vi "LoadHexaSummary1.vi"(7 "Machine":string, 10 "file path (dialog if empty)":path=path "C:/m300/HEXA/R141201634_20141222_141239.lot") -> (0 "error out":errorcluster)   [LabVIEW 2012]
uses:
  <vilib>/Utility/miscctls.llb/LVDateTimeRec.ctl
  <vilib>/addons/database/Auxilliary.llb/DB Tools Cursor Type.ctl
  <vilib>/addons/database/Connection.llb/DB Tools Open Connec (Path).vi
  <vilib>/addons/database/Connection.llb/Conn Execute.vi
  <vilib>/addons/database/Recordset.llb/Rec Fetch Integer Data (R).vi
  <vilib>/addons/database/Recordset.llb/Rec Destroy - Connection.vi
  <vilib>/addons/database/NI_Database_API.lvlib
panel:
  in  "Cluster 2":T1
  out "array":string[][](array[string])
  out "concatenated string":string
  in  "date time rec":T2
  in  "Cluster":T3
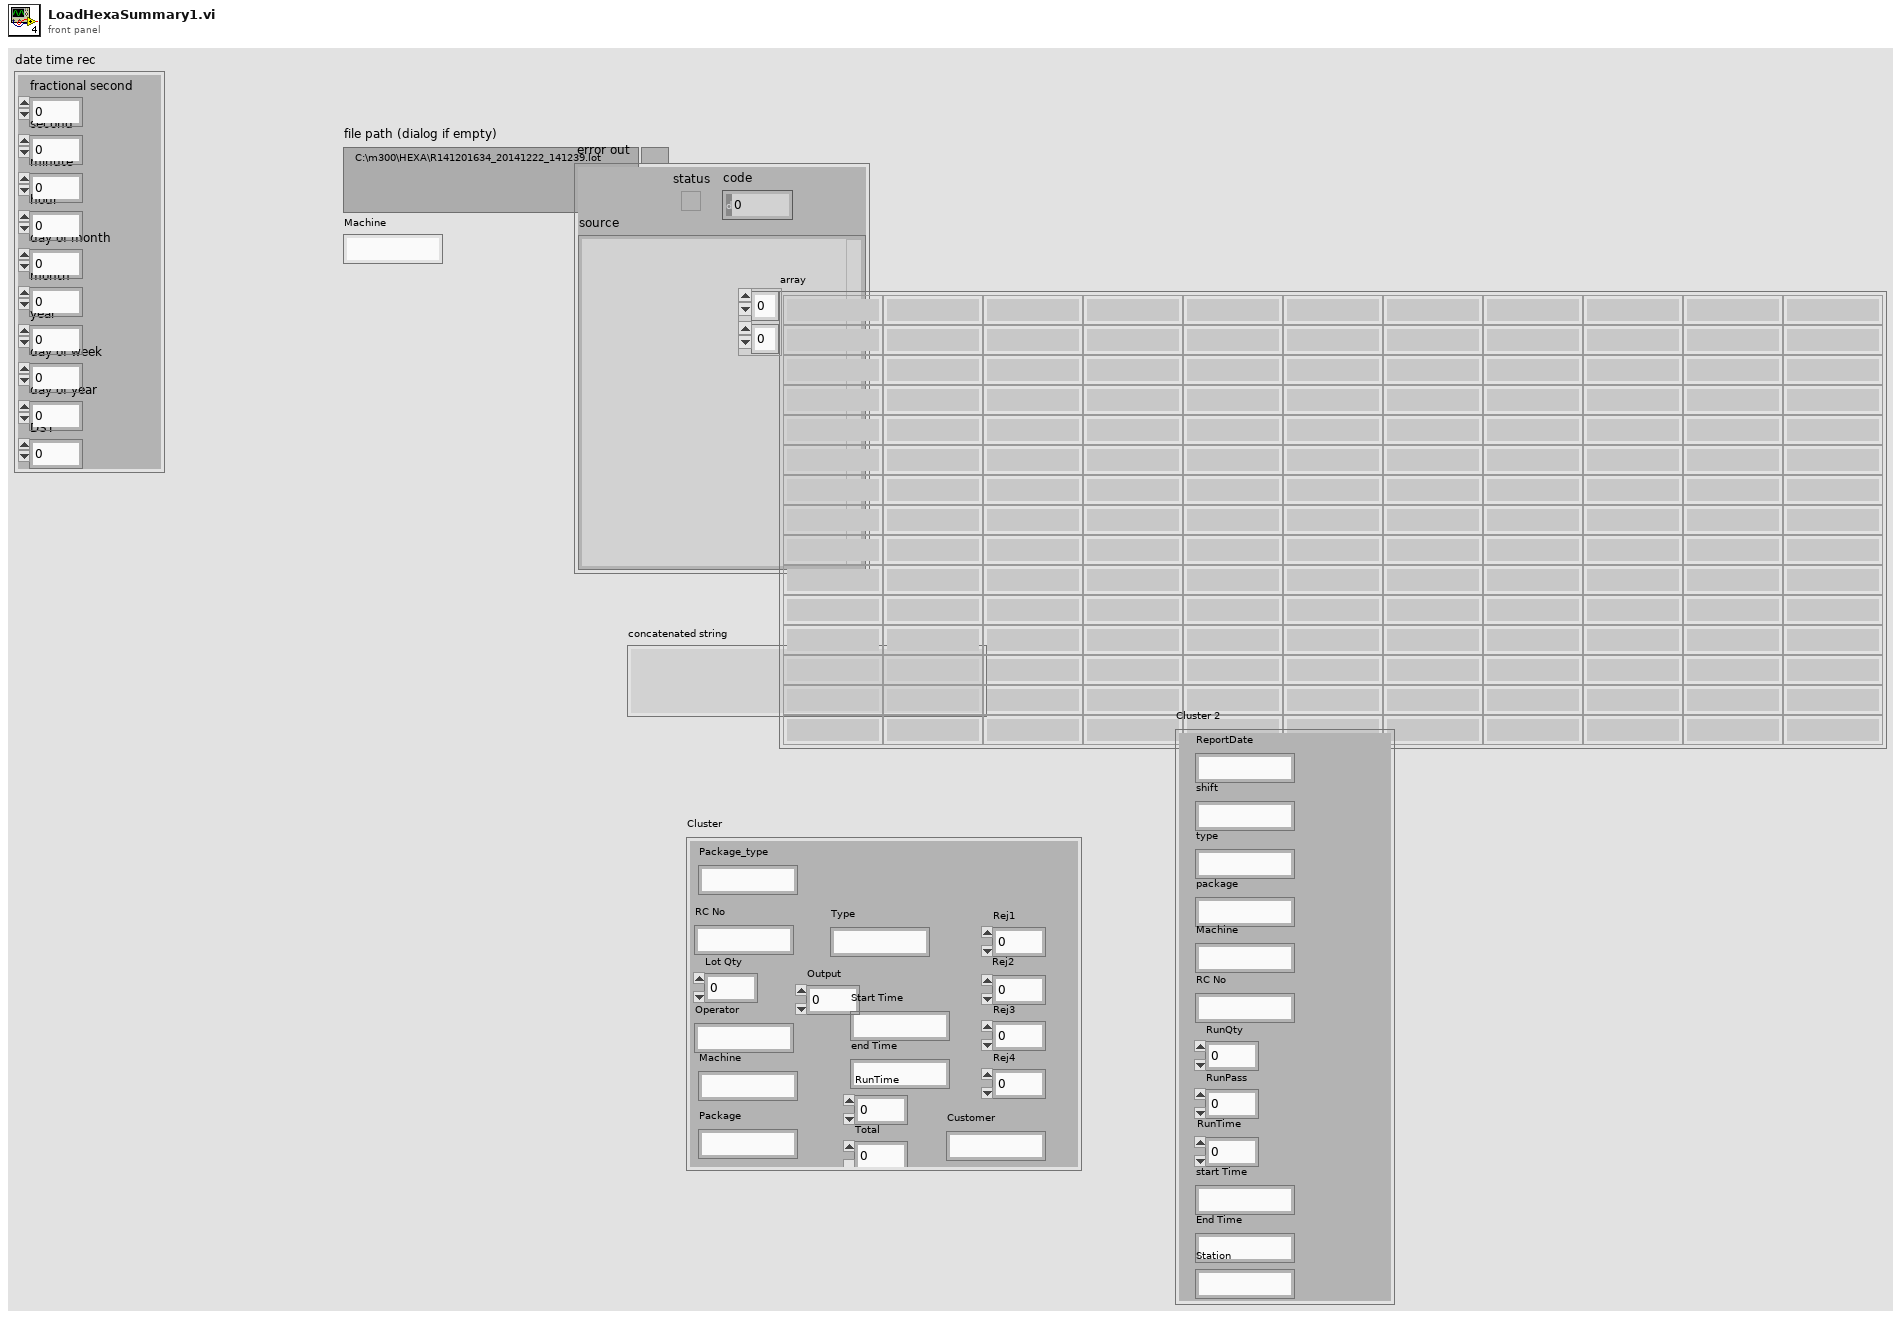
[diagram p1: front panel]
types:
  T1 = cluster{"ReportDate":string, "shift":string, "type":string, "package":string, "Machine":string, "RC No":string, "RunQty":dbl, "RunPass":dbl, "RunTime":dbl, "start Time":string, "End Time":string, "Station":string}
  T2 = typedef "LVDateTimeRec.ctl" = cluster{"fractional second":dbl, "second":i32, "minute":i32, "hour":i32, "day of month":i32, "month":i32, "year":i32, "day of week":i32, "day of year":i32, "DST":i32}
  T3 = cluster{"Package_type":string, "RC No":string, "Lot Qty":dbl, "Operator":string, "Machine":string, "Package":string, "Type":string, "Output":dbl, "Start Time":string, "end Time":string, "RunTime":dbl, "Total":dbl, "Rej1":dbl, "Rej2":dbl, "Rej3":dbl, "Rej4":dbl, "Customer":string}
  T4 = typedef "NI_Database_API.lvlib/DB Tools Cursor Type.ctl" = enum16{"forward-only", "keyset", "dynamic", "static"}
  T5 = typedef "NI_Database_API.lvlib/Conn ObjectReference.ctl" = refnum<k1>
  T6 = typedef "NI_Database_API.lvlib/Rec ObjectReference.ctl" = refnum<k1>
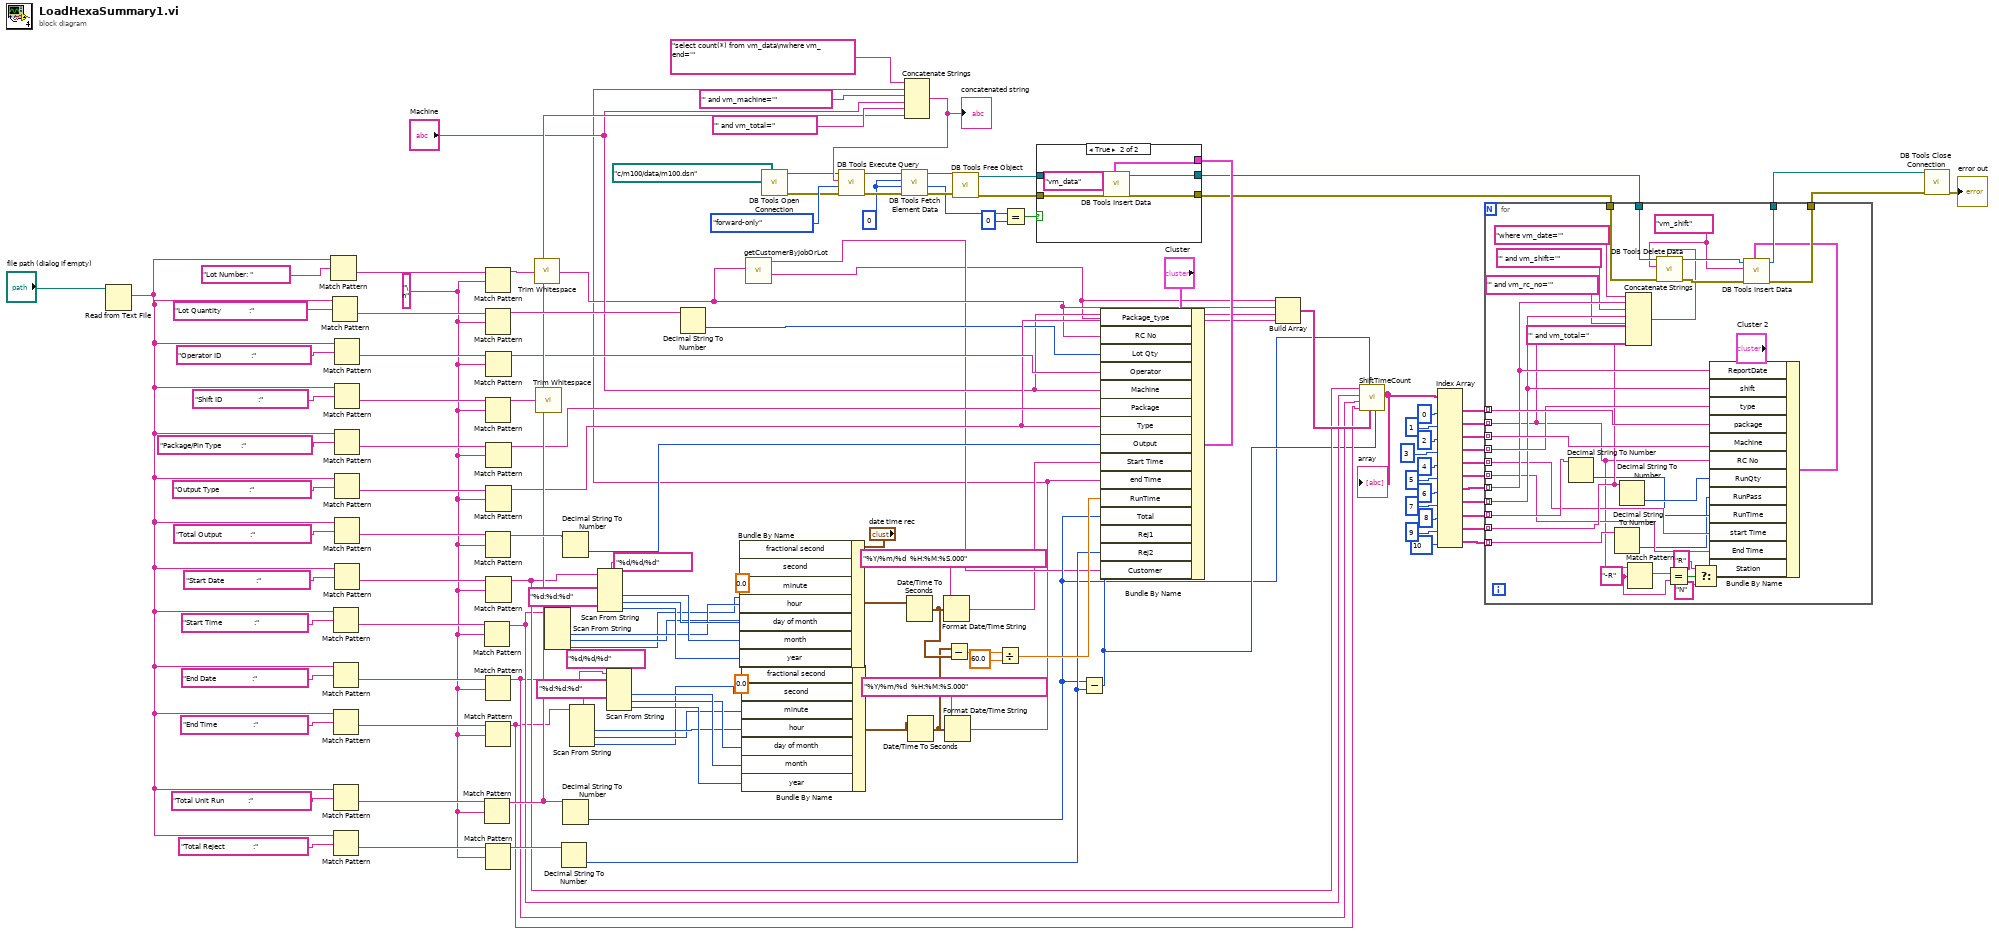
[diagram p0: block diagram]
diagram:
  w61 = 0
  w102 = "\n" ("regular expression")
  n1 = Read from Text File(file (use dialog)="file path (dialog if empty)") -> (text=w101:string)  [unwired: 3 in, 3 out]
  n2 = Match Pattern(string=w101, regular expression="Lot Number: ") -> (after substring=w127:string)  [unwired: 1 in, 3 out]
  n3 = Match Pattern(string=w101, regular expression="Lot Quantity              :") -> (after substring=w126:string)  [unwired: 1 in, 3 out]
  n4 = Match Pattern(string=w101, regular expression="Start Time                :") -> (after substring=w110:string)  [unwired: 1 in, 3 out]
  n5 = Match Pattern(string=w101, regular expression="End Date                  :") -> (after substring=w109:string)  [unwired: 1 in, 3 out]
  n6 = Match Pattern(string=w101, regular expression="End Time                  :") -> (after substring=w107:string)  [unwired: 1 in, 3 out]
  n7 = Match Pattern(string=w101, regular expression="Total Unit Run            :") -> (after substring=w104:string)  [unwired: 1 in, 3 out]
  n8 = Match Pattern(string=w101, regular expression="Total Reject              :") -> (after substring=w103:string)  [unwired: 1 in, 3 out]
  n9 = Match Pattern(string=w101, regular expression="Operator ID               :") -> (after substring=w123:string)  [unwired: 1 in, 3 out]
  n10 = Match Pattern(string=w101, regular expression="Shift ID                  :") -> (after substring=w120:string)  [unwired: 1 in, 3 out]
  n11 = Match Pattern(string=w101, regular expression="Package/Pin Type          :") -> (after substring=w119:string)  [unwired: 1 in, 3 out]
  n12 = Match Pattern(string=w101, regular expression="Output Type               :") -> (after substring=w117:string)  [unwired: 1 in, 3 out]
  n13 = Match Pattern(string=w101, regular expression="Total Output              :") -> (after substring=w114:string)  [unwired: 1 in, 3 out]
  n14 = Match Pattern(string=w101, regular expression="Start Date                :") -> (after substring=w113:string)  [unwired: 1 in, 3 out]
  n15 = Match Pattern(string=w110, regular expression=w102) -> (before substring=w38:string)  [unwired: 1 in, 3 out]
  n16 = Match Pattern(string=w104, regular expression=w102) -> (before substring=w47:string)  [unwired: 1 in, 3 out]
  n17 = Match Pattern(string=w127, regular expression=w102) -> (before substring=w54:string)  [unwired: 1 in, 3 out]
  n18 = Match Pattern(string=w126, regular expression=w102) -> (before substring=w125:string)  [unwired: 1 in, 3 out]
  n19 = Match Pattern(string=w120, regular expression=w102) -> (before substring=w53:string)  [unwired: 1 in, 3 out]
  n20 = Match Pattern(string=w114, regular expression=w102) -> (before substring=w100:string)  [unwired: 1 in, 3 out]
  n21 = Match Pattern(string=w109, regular expression=w102) -> (before substring=w37:string)  [unwired: 1 in, 3 out]
  n22 = Match Pattern(string=w107, regular expression=w102) -> (before substring=w36:string)  [unwired: 1 in, 3 out]
  n23 = Match Pattern(string=w103, regular expression=w102) -> (before substring=w72:string)  [unwired: 1 in, 3 out]
  n24 = Match Pattern(string=w123, regular expression=w102) -> (before substring=w45:string)  [unwired: 1 in, 3 out]
  n25 = Match Pattern(string=w119, regular expression=w102) -> (before substring=w46:string)  [unwired: 1 in, 3 out]
  n26 = Match Pattern(string=w117, regular expression=w102) -> (before substring=w44:string)  [unwired: 1 in, 3 out]
  n27 = Match Pattern(string=w113, regular expression=w102) -> (before substring=w39:string)  [unwired: 1 in, 3 out]
  n28 = call <vilib>:"Trim Whitespace.vi"("string"=w54) -> ("trimmed string"=w5:string)  [unwired: 1 in]
  n29 = call <vilib>:"Trim Whitespace.vi"("string"=w53) -> ()  [unwired: 1 in, 1 out]
  n30 = Scan From String(format string="%d:%d:%d", input string=w38) -> (output 1=w94:i32, output 2=w93:i32, output 3=w92:i32)  [unwired: 5 in, 3 out]
  n31 = Decimal String To Number(string=w72) -> (number=w70:i32)  [unwired: 2 in, 1 out]
  n32 = Decimal String To Number(string=w100) -> (number=w73:i32)  [unwired: 2 in, 1 out]
  n33 = Decimal String To Number(string=w47) -> (number=w6:i32)  [unwired: 2 in, 1 out]
  n34 = Scan From String(format string="%d:%d:%d", input string=w36) -> (output 1=w84:i32, output 2=w83:i32, output 3=w82:i32)  [unwired: 5 in, 3 out]
  n35 = Scan From String(format string="%d/%d/%d", input string=w39) -> (output 1=w98:i32, output 2=w97:i32, output 3=w96:i32)  [unwired: 5 in, 3 out]
  n36 = Scan From String(format string="%d/%d/%d", input string=w37) -> (output 1=w87:i32, output 2=w86:i32, output 3=w85:i32)  [unwired: 5 in, 3 out]
  n37 = Decimal String To Number(string=w125) -> (number=w41:i32)  [unwired: 2 in, 1 out]
  n38 = Bundle By Name(cluster="date time rec", "fractional second"=0.0, "second"=w92, "minute"=w93, "hour"=w94, "day of month"=w97, "month"=w98, "year"=w96) -> (w80:T2)
  n39 = Bundle By Name(cluster="date time rec", "fractional second"=0.0, "second"=w82, "minute"=w83, "hour"=w84, "day of month"=w86, "month"=w87, "year"=w85) -> (w77:T2)
  n40 = call "getCustomerByJobOrLot.vi"("Lot"=w5) -> ("Package"=w3:string, "CustomerID"=w4:string)  [unwired: 9 in]
  n41 = call-poly <vilib>:"DB Tools Open Connection.vi"("connection information"=path "c:/m100/data/m100.dsn") -> ("error out"=w50:errorcluster, "connection reference"=w51:T5)  [unwired: 7 in]
  n42 = Date/Time To Seconds(2:w80) -> (0:w43:timestamp)  [unwired: 1 in]
  n43 = Date/Time To Seconds(2:w77) -> (0:w42:timestamp)  [unwired: 1 in]
  n44 = Format Date/Time String(time format string (%c)="%Y/%m/%d  %H:%M:%S.000", seconds (now)=w43) -> (date/time string=w2:string)  [unwired: 1 in]
  n45 = Format Date/Time String(time format string (%c)="%Y/%m/%d  %H:%M:%S.000", seconds (now)=w42) -> (date/time string=w1:string)  [unwired: 1 in]
  n46 = Concatenate Strings("select count(*) from vm_data\nwhere vm_end='" ("SQL query"), w1, "' and vm_machine='" ("string"), "Machine", "' and vm_total=" ("string"), w47) -> (w52:string)
  "concatenated string" <- w52
  n47 = call-poly <vilib>:"DB Tools Execute Query.vi"("error in (no error)"=w50, "cursor type"=DB_Tools_Cursor_Type."forward-only", "SQL query"=w52, "connection reference"=w51) -> ("error out"=w67:errorcluster, "recordset reference"=w69:T6)  [unwired: 4 in]
  n48 = call-poly <vilib>:"DB Tools Fetch Element Data.vi"("error in (no error)"=w67, "type"=w61, "column index"=w61, "recordset reference"=w69) -> ("error out"=w66:errorcluster, "data"=w60:i32, "recordset reference out"=w68:T6)  [unwired: 3 in]
  n49 = Subtract(x=w42, y=w43) -> (x-y=w76:dbl)
  n50 = call-poly <vilib>:"DB Tools Free Object.vi"("error in (no error)"=w66, "recordset reference"=w68) -> ("error out"=w56:errorcluster, "connection reference"=w57:T5)  [unwired: 8 in]
  n51 = Divide(x=w76, y=60.0) -> (x/y=w71:dbl)
  n52 = Equal?(x=w60, y=0) -> (x = y?=w58:bool)
  n53 = Subtract(x=w6, y=w70) -> (x-y=w7:i32)
  n54 = Bundle By Name(cluster="Cluster", "Package_type"=w3, "RC No"=w5, "Lot Qty"=w41, "Operator"=w45, "Machine"="Machine", "Package"=w46, "Type"=w44, "Output"=w73, "Start Time"=w2, "end Time"=w1, "RunTime"=w71, "Total"=w6, "Rej1"=w7, "Rej2"=w70, "Customer"=w4) -> (w55:T3)
  n55 = case shown="True" w58 {
    tunnel: w57 -> [w132 w138]
    tunnel: w56 -> [w131 w137]
    tunnel: [w132 w136] -> w13
    tunnel: [w131 w135] -> w12
    tunnel: w55 -> [_ w134]
    frame False {
    }
    frame True {
      n56 = call <vilib>:"DB Tools Insert Data.vi"("data"=w134, "error in (no error)"=w137, "table"="vm_data", "connection reference"=w138) -> ("error out"=w135:errorcluster, "connection reference out"=w136:T5)  [unwired: 6 in]
    }
  }
  n57 = Build Array(w3, w5, "Machine", w44) -> (w40:string[])
  n58 = call "ShiftTimeCount.vi"("PASS"=w7, "BasicData"=w40, "Qty"=w6, "EndTime 2"=w36, "date string"=w37, "BegTime"=w38, "BegDate"=w39) -> ("array"=w34:string[][])  [unwired: 4 in]
  "array" <- w34
  n59 = Index Array(array=w34, index (col) #1=0 ("disabled index (col)"), index (col) #2=1 ("index (col)"), index (col) #3=2 ("index (col)"), index (col) #4=3 ("index (col)"), index (col) #5=4 ("index (col)"), index (col) #6=5 ("index (col)"), index (col) #7=6 ("index (col)"), index (col) #8=7 ("index (col)"), index (col) #9=8 ("index (col)"), index (col) #10=9 ("index (col)"), index (col) #11=10 ("index (col)")) -> (element #1=w23:string[], element #2=w22:string[], element #3=w21:string[], element #4=w20:string[], element #5=w19:string[], element #6=w18:string[], element #7=w17:string[], element #8=w16:string[], element #9=w15:string[], element #10=w14:string[], element #11=w8:string[])  [unwired: 11 in]
  n60 = for {
    tunnel: w23 -> [w171] mode=indexing
    tunnel: w22 -> [w145] mode=indexing
    tunnel: w21 -> [w170] mode=indexing
    tunnel: w20 -> [w169] mode=indexing
    tunnel: w19 -> [w149] mode=indexing
    tunnel: w18 -> [w150] mode=indexing
    tunnel: w17 -> [w156] mode=indexing
    tunnel: w16 -> [w154] mode=indexing
    tunnel: w15 -> [w168] mode=indexing
    tunnel: w14 -> [w151] mode=indexing
    tunnel: w13 -> [w161]
    tunnel: w12 -> [w160]
    tunnel: [w166] -> w11
    tunnel: [w165] -> w10
    tunnel: w8 -> [w146] mode=indexing
    w143 = "-R" ("regular expression")
    w159 = "vm_shift" ("table")
    n61 = Decimal String To Number(string=w168) -> (number=w148:i32)  [unwired: 2 in, 1 out]
    n62 = Decimal String To Number(string=w146) -> (number=w147:i32)  [unwired: 2 in, 1 out]
    n63 = Decimal String To Number(string=w151) -> (number=w167:i32)  [unwired: 2 in, 1 out]
    n64 = Concatenate Strings("where vm_date='" ("string"), w156, "' and vm_shift='" ("string"), w154, "' and vm_rc_no='" ("string"), w145, "' and vm_total=" ("string"), w151) -> (w158:string)
    n65 = Match Pattern(string=w145, regular expression=w143) -> (match substring=w144:string)  [unwired: 1 in, 3 out]
    n66 = call <vilib>:"DB Tools Delete Data.vi"("condition"=w158, "error in (no error)"=w160, "table"=w159, "connection reference"=w161) -> ("error out"=w162:errorcluster, "connection reference out"=w163:T5)  [unwired: 6 in]
    n67 = Equal?(x=w144, y=w143) -> (x = y?=w142:bool)
    n68 = Select(t="R", s=w142, f="N") -> (s? t:f=w139:string)
    n69 = Bundle By Name(cluster="Cluster 2", "ReportDate"=w156, "shift"=w154, "type"=w169, "package"=w171, "Machine"=w170, "RC No"=w145, "RunQty"=w167, "RunPass"=w147, "RunTime"=w148, "start Time"=w149, "End Time"=w150, "Station"=w139) -> (w164:T1)
    n70 = call <vilib>:"DB Tools Insert Data.vi"("data"=w164, "error in (no error)"=w162, "table"=w159, "connection reference"=w163) -> ("error out"=w165:errorcluster, "connection reference out"=w166:T5)  [unwired: 6 in]
  }
  n71 = call <vilib>:"DB Tools Close Connection.vi"("error in (no error)"=w10, "connection reference"=w11) -> ("error out"=→"error out":errorcluster)  [unwired: 5 in]
